vi "FindLocation_SingleAxis.vi"(4 "error in (no error)":errorcluster, 6 "Axis (0 is X)":i32, 7 "Motion Settings":T1={"No Motion?"=FALSE, "Motion System"=enum."NI 735x", "Motion Bd ID"=1, "Motion Profile"="SMAC1", "# Axis"=1, "Reverse Z axis?"=TRUE, "SMAC Axis"=0, "scan pair"=enum."y-(x) scan", "RT fps"=6.0, "Steps per mm"=[1000, 1000, 1000, 1000], "Motor Parameters"={"velocity ct/s"=[10000.0, 10000.0, 10000.0, 50000.0], "accel ct/s^2"=[50000.0, 50000.0, 50000.0, 200000.0]}, "One Way Scan"=FALSE, "Reverse One Way Scan"=FALSE, "Global Position (mm)"=[], "Plane"=0, "Distance between\nscan lines (um)"=0.0, "Distance between\nscan planes (um)"=0.0, "number of scan planes"=1, "Total steps in line"=0, "Xtra plane\ndistance  (um)"=100, "Xtra planes "=1, "Add Axis"=FALSE, "overshoot cts"=200, "BKPT Shift"=0, "Scan Start Time (ms)"=0, "ESP VISA"="GPIB::1::INSTR", "3rd Axis"=1, "GL Ref Out"=refnum, "Galil Address"=""} {"3rd Axis" items=["x", "y", "z", "w"]; "Xtra planes" min=1; "Xtra plane\ndistance  (um)" min=0; "Distance between\nscan planes (um)" format="%.2f"; "Distance between\nscan lines (um)" format="%.2f"; "SMAC Axis" items=["None"=0, "Axis 1"=1, "Axis 2"=2, "Axis 3"=3, "Axis 4"=4, "Axis 5"=5, "Axis 6"=6, "Axis 7"=7, "Axis 8"=8, "Vector Space 1"=17, "Vector Space 2"=18, "Vector Space 3"=19, "Vector Space 4"=20]; "Motion Bd ID" min=1 max=32 step=1}) -> (0 "error out":errorcluster, 1 "Global Position":dbl[](array[numeric]), 2 "Position (mm) (Abs)":dbl format="%.3f", 3 "Bd ID Out":u8)   [LabVIEW 2022 SP3]
uses:
  MotionParameters.ctl
  MotionSys.ctl
  -MotionRoutines/ScanAxis.ctl
  -MotionRoutines/3rdAxis.ctl
panel:
  # "1-D and 2-D B scan settings"
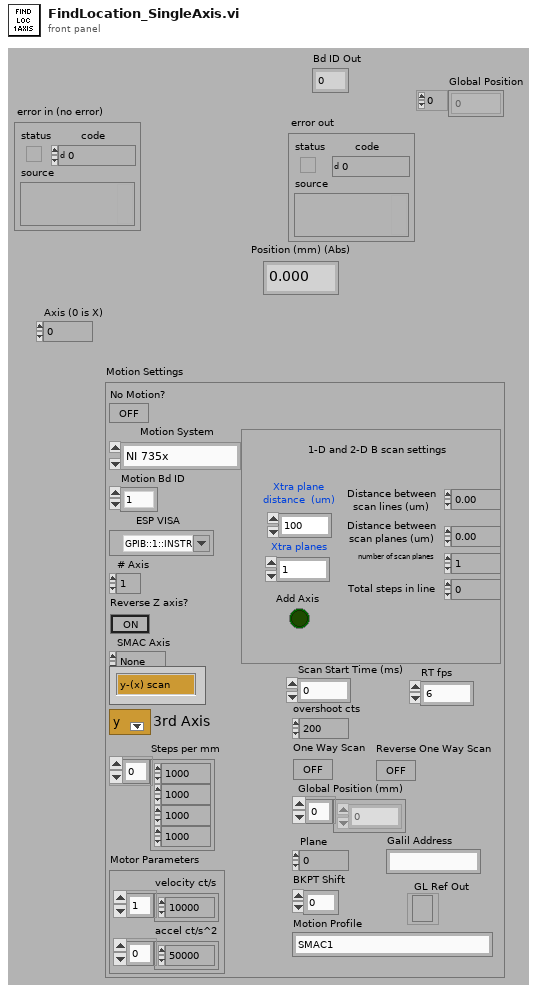
[diagram p1: front panel]
types:
  T1 = typedef "MotionParameters.ctl" = cluster{"No Motion?":bool, "Motion System":T2, "Motion Bd ID":u8, "Motion Profile":string, "# Axis":i8, "Reverse Z axis?":bool, "SMAC Axis":u16, "scan pair":T3, "RT fps":sgl, "Steps per mm":i32[], "Motor Parameters":cluster{"velocity ct/s":dbl[], "accel ct/s^2":dbl[]}, "One Way Scan":bool, "Reverse One Way Scan":bool, "Global Position (mm)":dbl[], "Plane":i32, "Distance between\nscan lines (um)":sgl, "Distance between\nscan planes (um)":sgl, "number of scan planes":i32, "Total steps in line":i32, "Xtra plane\ndistance  (um)":i32, "Xtra planes ":i32, "Add Axis":bool, "overshoot cts":i32, "BKPT Shift":i32, "Scan Start Time (ms)":u32, "ESP VISA":refnum<visa-resource-name>, "3rd Axis":T4, "GL Ref Out":refnum<k7>, "Galil Address":string}
  T2 = typedef "MotionSys.ctl" = enum16{"MM3000", "NI 735x", "Newport ESP", "No Motion Card", "Galil"}
  T3 = typedef "ScanAxis.ctl" = enum16{"y-(x) scan", "x-(y) scan", "z-(x) scan", "z-(y) scan", "y-(z) scan", "x-(z) scan", "w-(x) scan", "w-(y) scan", "w-(z) scan", "x-(w) scan", "y-(w) scan", "z-(w) scan"}
  T4 = typedef "3rdAxis.ctl" = u16
  T5 = cluster{"Reserved":bool, "Axis #1 Move Complete":bool, "Axis #2 Move Complete":bool, "Axis #3 Move Complete":bool, "Axis #4 Move Complete":bool, "Axis #5 Move Complete":bool, "Axis #6 Move Complete":bool, "Axis #7 Move Complete":bool, "Axis #8 Move Complete":bool, "Axis #9 MoveComplete":bool, "Axis #10 Move Complete":bool, "Axis #11 Move Complete":bool, "Axis #12 Move Complete":bool, "Status #13":bool, "Status #14":bool, "Status #15":bool}
  T6 = typedef "Bd Id Out" = u8
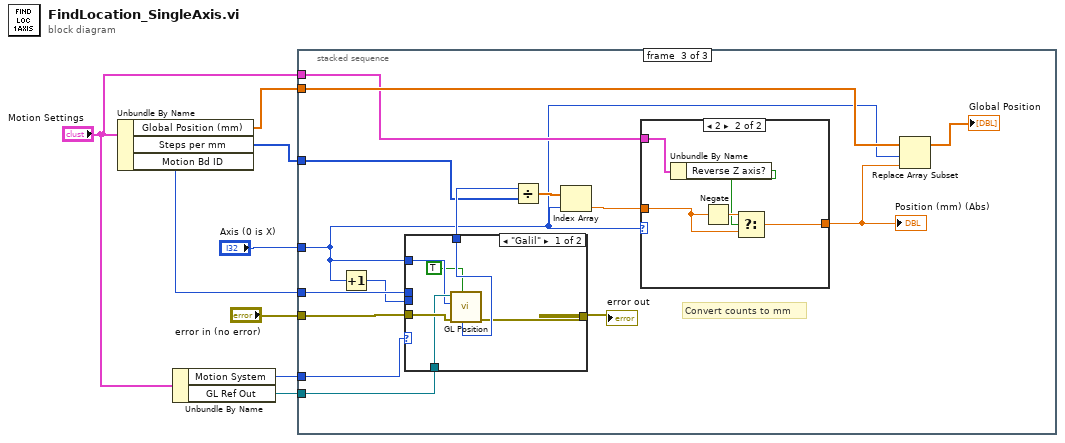
[diagram p0: block diagram]
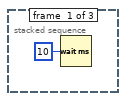
[diagram p2: hidden frame]
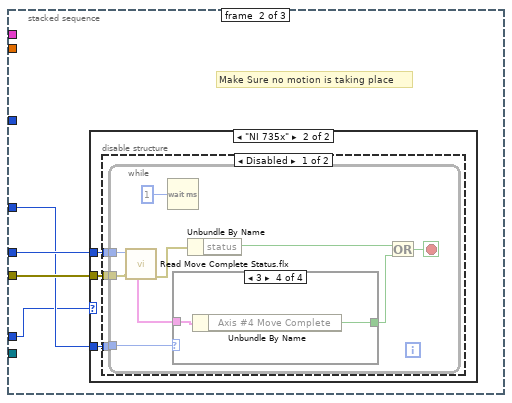
[diagram p3: hidden frame]
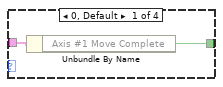
[diagram p5: hidden frame]
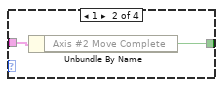
[diagram p6: hidden frame]
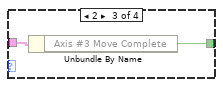
[diagram p7: hidden frame]
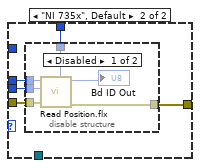
[diagram p9: hidden frame]
diagram:
  n1 = Unbundle By Name("Motion Settings") -> ("Global Position (mm)"=w5:dbl[], "Steps per mm"=w6:i32[], "Motion Bd ID"=w4:u8)
  n2 = Unbundle By Name("Motion Settings") -> ("Motion System"=w2:T2, "GL Ref Out"=w1:refnum<k7>)
  n3 = stacked-sequence {
    tunnel: "error in (no error)" -> [_ w12 w49]
    tunnel: w4 -> [_ w13 w48]
    tunnel: "Axis (0 is X)" -> [_ w11 w37]
    tunnel: w6 -> [_ _ w42]
    tunnel: w5 -> [_ _ w41]
    tunnel: "Motion Settings" -> [_ _ w40]
    tunnel: w2 -> [_ w10 w39]
    tunnel: w1 -> [_ _ w38]
    frame #0 {
      n4 = Wait (ms)(milliseconds to wait=10) -> ()  [unwired: 1 out]
    }
    frame #1 {
      # "Make Sure no motion is taking place"
      n5 = case shown="\"NI 735x\"" w10 {
        tunnel: w13 -> [_ w16]
        tunnel: w12 -> [_ w15]
        tunnel: w11 -> [_ w14]
        frame "Galil", Default {
        }
        frame "NI 735x" {
          n6 = disable-structure shown="Disabled" {
            disable-tunnel: w16 -> [w19 _]
            disable-tunnel: w15 -> [w18 _]
            disable-tunnel: w14 -> [w17 _]
            frame Disabled {
              n7 = while {
                tunnel: w19 -> [w28]
                tunnel: w18 -> [w22]
                tunnel: w17 -> [w21]
                stop <- w24 stop-if-true
                n8 = call <vilib>:"Read Move Complete Status.flx"("error in (no error)"=w22, "Board ID"=w28) -> ("error out"=w20:errorcluster, "Move Complete Status"=w27:T5)  [unwired: 1 in, 4 out]
                n9 = Wait (ms)(milliseconds to wait=1) -> ()  [unwired: 1 out]
                n10 = case shown="3" w21 {
                  tunnel: w27 -> [w30 w32 w34 w36]
                  tunnel: [w29 w31 w33 w35] -> w25
                  frame 0, Default {
                    n11 = Unbundle By Name(w30) -> ("Axis #1 Move Complete"=w29:bool)
                  }
                  frame 1 {
                    n12 = Unbundle By Name(w32) -> ("Axis #2 Move Complete"=w31:bool)
                  }
                  frame 2 {
                    n13 = Unbundle By Name(w34) -> ("Axis #3 Move Complete"=w33:bool)
                  }
                  frame 3 {
                    n14 = Unbundle By Name(w36) -> ("Axis #4 Move Complete"=w35:bool)
                  }
                }
                n15 = Unbundle By Name(w20) -> ("status"=w26:bool)
                n16 = Or(x=w26, y=w25) -> (x .or. y?=w24:bool)
              }
            }
            frame Enabled {
            }
          }
        }
      }
    }
    frame #2 {
      # "Convert counts to mm"
      n17 = Increment(x=w37) -> (x+1=w46:i32)
      n18 = case shown="\"Galil\"" w39 {
        tunnel: [w56 w62] -> w51
        tunnel: [w57 w61] -> w50
        tunnel: w49 -> [w55 w60]
        tunnel: w48 -> [_ w59]
        tunnel: w46 -> [_ w58]
        tunnel: w38 -> [w54 _]
        tunnel: w37 -> [w53 _]
        frame "Galil" {
          n19 = call "GL Position.vi"("Wait for Motion Complete"=TRUE, "error in (no error)"=w55, "Axis"=w53, "Galil.IGalil"=w54) -> ("error out"=w56:errorcluster, "Axis Position"=w57:i32)  [unwired: 2 in, 2 out]
        }
        frame "NI 735x", Default {
          n20 = disable-structure shown="Disabled" {
            disable-tunnel: [w68 _] -> w62
            disable-tunnel: [w67 _] -> w61
            disable-tunnel: w60 -> [w66 _]
            disable-tunnel: w59 -> [w65 _]
            disable-tunnel: w58 -> [w64 _]
            frame Disabled {
              n21 = call <vilib>:"Read Position.flx"("error in (no error)"=w66, "Axis"=w64, "Board ID"=w65) -> ("error out"=w68:errorcluster, "Bd ID Out"=→"Bd ID Out":T6, "Position"=w67:i32)  [unwired: 4 out]
            }
            frame Enabled {
            }
          }
        }
      }
      "error out" <- w51
      n22 = Divide(x=w50, y=w42) -> (x/y=w47:dbl[])
      n23 = Index Array(array=w47, index=w37) -> (element=w45:dbl)
      n24 = case shown="2" w37 {
        tunnel: w45 -> [w69 w73]
        tunnel: [w69 w72] -> w43
        tunnel: w40 -> [_ w71]
        frame 0, Default {
        }
        frame 2 {
          n25 = Unbundle By Name(w71) -> ("Reverse Z axis?"=w70:bool)
          n26 = Negate(x=w73) -> (-x=w74:dbl)
          n27 = Select(t=w74, s=w70, f=w73) -> (s? t:f=w72:dbl)
        }
      }
      "Position (mm) (Abs)" <- w43
      n28 = Replace Array Subset(array=w41, new element=w43, index=w37) -> (→"Global Position":dbl[])
    }
  }
